vi "SSC DCPower Debug Global.vi"() -> ()   [LabVIEW 2020]
uses:
  <instrlib>/niDCPower/nidcpower.llb/niDCPower Power Line Frequency.ctl
panel:
  in  "power line frequency":T1=60.0 items=["50 Hertz"=50.0, "60 Hertz"=60.0]
  in  "Measure Multiple Only?":bool
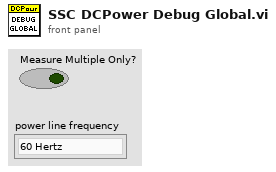
[diagram p1: front panel]
types:
  T1 = typedef "niDCPower Power Line Frequency.ctl" = dbl
diagram:
